vi "MutliVu Interface Test.vi"() -> ()   [LabVIEW 2020]
panel:
  out "Field\nStatus":i32(ring)=4 items=["MagnetUnknown"=0, "StablePersistent"=1, "WarmingSwitch"=2, "CoolingSwitch"=3, "StableDriven"=4, "Iterating"=5, "Charging"=6, "Discharging"=7, "CurrentError"=8, "MagnetFailure"=15]
  out "Temperature\nStatus":i32(ring)=1 items=["TemperatureUnknown"=0, "Stable"=1, "Tracking"=2, "Near"=5, "Chasing"=6, "Filling"=7, "Standby"=10, "Disabled"=13, "ImpedanceNotFunction"=14, "TempFailure"=15]
  out "Chamber\nStatus":i32(ring)=3 items=["ChamberUnknown"=0, "PurgedAndSealed"=1, "VentedAndSealed"=2, "Sealed"=3, "Purging"=4, "Venting"=5, "PreHiVac"=6, "HighVac"=7, "PumpContinuous"=8, "VentContinuous"=9, "ChamberFailure"=15]
  out "Initialised":bool=TRUE
  in  "stop":bool
  in  "Set Chamber":bool caption="Set Temperature"
  in  "Set Position":bool caption="Set Temperature"
  in  "Set Field":bool caption="Set Temperature"
  in  "Set Temperature":bool
  in  "Chamber Setpoint":i32(ring)=1 caption="Chamber" items=["Seal", "PurgeAndSeal", "VentAndSeal", "PumpContinuous", "VentContinuous", "HighVacuum"]
  out "Position":dbl=1.80066852665739e-41
  in  "Position Setpoint":dbl caption="Position (degrees)" min=-10.0 max=370.0
  out "Field":dbl=0.3983127772808075
  out "Temperature":dbl=299.9980773925781
  in  "Field Setpoint":dbl caption="Field (Oe)" min=-90000.0 max=90000.0
  in  "temperature setpoint":dbl=300.0 caption="Temperature (K)" min=1.8 max=400.0
  in  "InstrumentType":i32(ring)=2 items=["PPMS", "VersaLab", "DynaCool", "SVSM", "OptiCool"]
  in  "Remote \nMode":bool
  in  "IP Address":string="10.29.163.8"
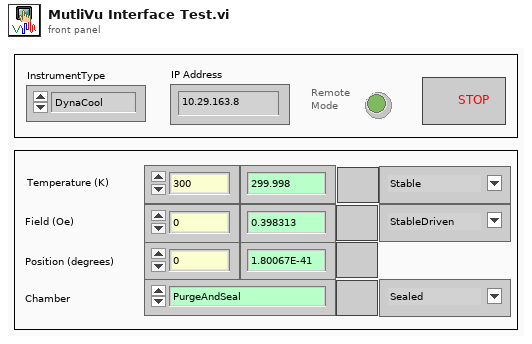
[diagram p1: front panel]
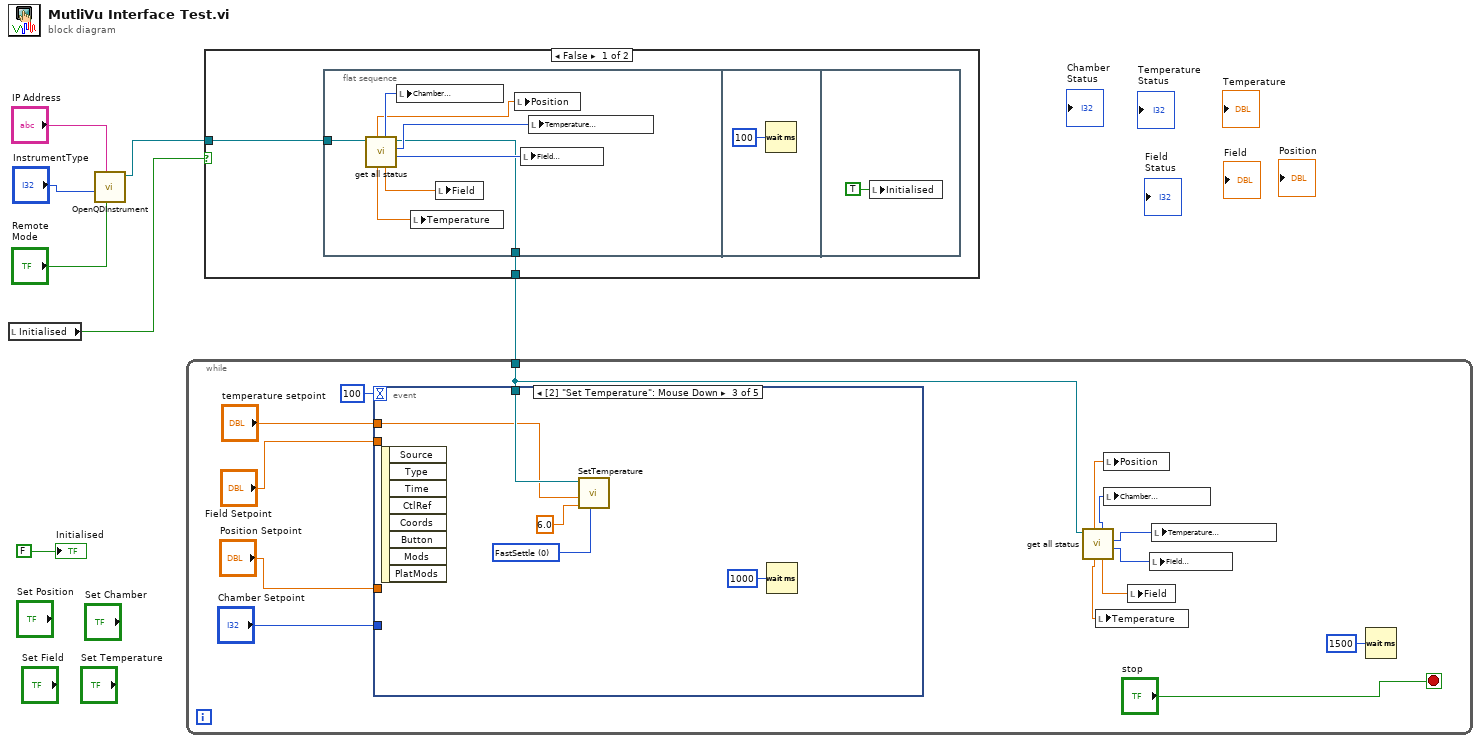
[diagram p0: block diagram]
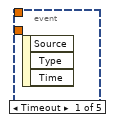
[diagram p3: hidden frame]
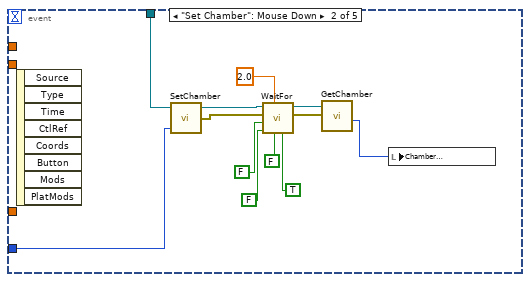
[diagram p4: hidden frame]
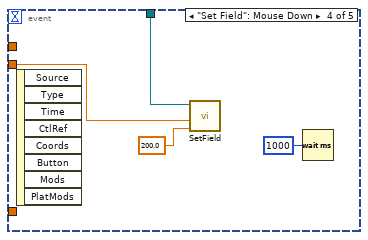
[diagram p5: hidden frame]
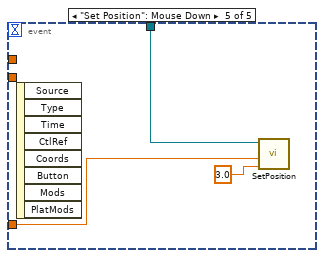
[diagram p6: hidden frame]
diagram:
  n1 = local read "Initialised"() -> (w3:bool)
  n2 = call "OpenQDInstrument.vi"("Remote"="Remote \nMode", "IP Address"="IP Address", "InstrumentType"="InstrumentType") -> ("Instrument Ref"=w2:refnum<k24>)  [unwired: 5 in, 1 out]
  n3 = case shown="False" w3 {
    tunnel: w2 -> [w9 w20]
    tunnel: [w8 w20] -> w1
    frame False {
      n4 = flat-sequence {
        tunnel: w9 -> [w17]
        tunnel: [w11] -> w8
        frame #0 {
          n5 = call "get all status.vi"("Instrument Ref In"=w17) -> ("Field\nStatus"=w14:i32, "Temperature\nStatus"=w15:i32, "Instrument Ref Out"=w11:refnum<k24>, "Field"=w12:dbl, "Chamber\nStatus"=w16:i32, "Temperature"=w13:dbl, "Position"=w10:dbl)  [unwired: 3 in, 1 out]
          n6 = local write "Chamber\nStatus"(w16) -> ()
          n7 = local write "Temperature"(w13) -> ()
          n8 = local write "Field"(w12) -> ()
          n9 = local write "Position"(w10) -> ()
          n10 = local write "Field\nStatus"(w14) -> ()
          n11 = local write "Temperature\nStatus"(w15) -> ()
        }
        frame #1 {
          n12 = Wait (ms)(milliseconds to wait=u32 100) -> ()  [unwired: 1 out]
        }
        frame #2 {
          n13 = local write "Initialised"(TRUE ("Initialised")) -> ()
        }
      }
    }
    frame True {
    }
  }
  n14 = while {
    tunnel: w1 -> [w23]
    stop <- "stop" stop-if-true
    n15 = event shown="[2] \"Set Temperature\": Mouse Down" {
      selector: _ -> [_ _ _ _ _]
      dyn-events: _ -> [_ _ _ _ _]
      timeout: 100 -> [_ _ _ _ _]
      tunnel: "Chamber Setpoint" -> [_ w46 _ _ _]
      tunnel: w23 -> [_ w45 w51 w54 w56]
      tunnel: "temperature setpoint" -> [_ _ w48 _ _]
      tunnel: "Field Setpoint" -> [_ _ _ w53 _]
      tunnel: "Position Setpoint" -> [_ _ _ _ w57]
      event Timeout {
        n16 = event-data() -> ()  [unwired: 1 in, 3 out]
      }
      event "Set Chamber": Mouse Down {
        n17 = event-data() -> ()  [unwired: 1 in, 8 out]
        n18 = call "SetChamber.vi"("Code"=w46, "Instrument Ref In"=w45) -> ("error out"=w36:errorcluster, "Instrument Ref Out"=w44:refnum<k24>)  [unwired: 1 in, 1 out]
        n19 = call "WaitFor.vi"("Wait For Chamber"=TRUE, "Wait For Position"=FALSE, "Delay"=2.0, "Wait For Field"=FALSE, "Wait For Temperature"=FALSE, "error in (no error)"=w36, "Instrument Ref In"=w44) -> ("error out"=w35:errorcluster, "Instrument Ref Out"=w39:refnum<k24>)  [unwired: 3 in]
        n20 = call "GetChamber.vi"("error in (no error)"=w35, "Instrument Ref In"=w39) -> ("Chamber\nStatus"=w38:i32)  [unwired: 2 in, 3 out]
        n21 = local write "Chamber\nStatus"(w38) -> ()
      }
      event "Set Temperature": Mouse Down {
        w49 = 0 items=["FastSettle", "NoOvershoot"] ("Approach")
        n22 = event-data() -> ()  [unwired: 1 in, 8 out]
        n23 = call "SetTemperature.vi"("Approach"=w49, "Rate"=6.0, "Temperature"=w48, "Instrument Ref In"=w51) -> ()  [unwired: 3 in, 3 out]
        n24 = Wait (ms)(milliseconds to wait=u32 1000) -> ()  [unwired: 1 out]
      }
      event "Set Field": Mouse Down {
        n25 = event-data() -> ()  [unwired: 1 in, 8 out]
        n26 = call "SetField.vi"("Rate"=200.0, "Field"=w53, "Instrument Ref In"=w54) -> ()  [unwired: 4 in, 3 out]
        n27 = Wait (ms)(milliseconds to wait=u32 1000) -> ()  [unwired: 1 out]
      }
      event "Set Position": Mouse Down {
        n28 = event-data() -> ()  [unwired: 1 in, 8 out]
        n29 = call "SetPosition.vi"("Speed"=3.0, "Position"=w57, "Instrument Ref In"=w56) -> ()  [unwired: 4 in, 3 out]
      }
    }
    n30 = call "get all status.vi"("Instrument Ref In"=w23) -> ("Field\nStatus"=w27:i32, "Temperature\nStatus"=w26:i32, "Field"=w29:dbl, "Chamber\nStatus"=w25:i32, "Temperature"=w28:dbl, "Position"=w22:dbl)  [unwired: 3 in, 2 out]
    n31 = local write "Temperature"(w28) -> ()
    n32 = local write "Position"(w22) -> ()
    n33 = local write "Chamber\nStatus"(w25) -> ()
    n34 = local write "Field"(w29) -> ()
    n35 = local write "Field\nStatus"(w27) -> ()
    n36 = local write "Temperature\nStatus"(w26) -> ()
    n37 = Wait (ms)(milliseconds to wait=u32 1500) -> ()  [unwired: 1 out]
  }
  "Initialised" <- FALSE ("Initialised")
